vi "Desonatter bezzer.vi"(10 "OK":bool) -> (2 "Array":bool[](array[boolean]))   [LabVIEW 2015]
uses:
  Galobal variable_TI.vi
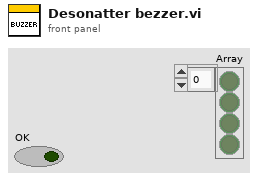
[diagram p1: front panel]
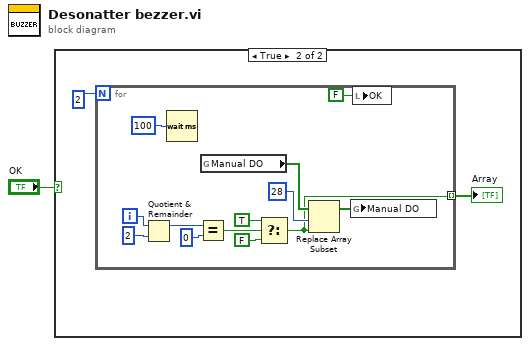
[diagram p0: block diagram]
diagram:
  n1 = case shown="True" "OK" {
    frame False {
    }
    frame True {
      n2 = for {
        N: 2 -> [_]
        tunnel: [w6] -> w2 mode=indexing
        i -> [w14]
        n3 = Quotient & Remainder(x=w14, y=2) -> (x-y*floor(x/y)=w12:i32)  [unwired: 1 out]
        n4 = Wait (ms)(milliseconds to wait=u32 100) -> ()  [unwired: 1 out]
        n5 = Equal?(x=w12, y=0) -> (x = y?=w10:bool)
        n6 = global read "Galobal variable_TI.vi" "Manual DO"() -> (w16:bool[])
        n7 = Select(t=TRUE, s=w10, f=FALSE) -> (s? t:f=w6:bool)
        n8 = Replace Array Subset(array=w16, new element=w6, index=28) -> (w7:bool[])
        n9 = global write "Galobal variable_TI.vi" "Manual DO"(w7) -> ()
        n10 = local write "OK"(FALSE ("OK")) -> ()
      }
      "Array" <- w2
    }
  }
